vi "SS_fpga_swept_sines.vi"() -> ()   [LabVIEW 2017]
uses:
  controls/boolean_info.ctl
  subVIs/auto-sys-id/controls/sysID_control_params.ctl
  <vilib>/rvi/Emulation/niFpgaGetClockAttributes.vi
  <vilib>/rvi/Emulation/niFpgaSctlEmulationGetInTimedLoop.vi
  <vilib>/rvi/Emulation/niFpgaEmulationReportErrorSimple.vi
  <vilib>/rvi/Emulation/niFpgaCriticalErrorInLSC.vi
  <vilib>/rvi/Emulation/niFpgaProcessEmulError.vi
panel:
  in  "Log-Channel_select":bool[](array[boolean])=[TRUE, TRUE, TRUE, TRUE, FALSE, FALSE]
  in  "Close Loop?":bool
  in  "Nsettle":u32
  in  "reset":bool=TRUE
  out "z-u(k)":sgl
  in  "DDS_params":T1={"Accumulator Increment"=100000, "Phase Shift"=0, "Signal Amplitude (x 2^15)"=32768}
  in  "DAC-select":i16(ring) items=["Mod2/AO0", "Mod2/AO1", "Mod2/AO2", "Mod2/AO3", ""]
  in  "ADC-select":i16(ring) items=["Mod2/AI0", "Mod2/AI1", "Mod2/AI2", "Mod2/AI3", ""]
  in  "ABORT":bool
  in  "Subtract y0?":bool
  in  "Swept-Sines-Control-Settings":T2={"u-max"=0.3, "offset"=0.0, "Ki"=0.001} {"offset" format="%#_4g"; "u-max" format="%#_13g"}
  out "iter":i32
  out "All Done":bool
  in  "TsTicks":u32=1600
  out "boolean \nindicators":T3
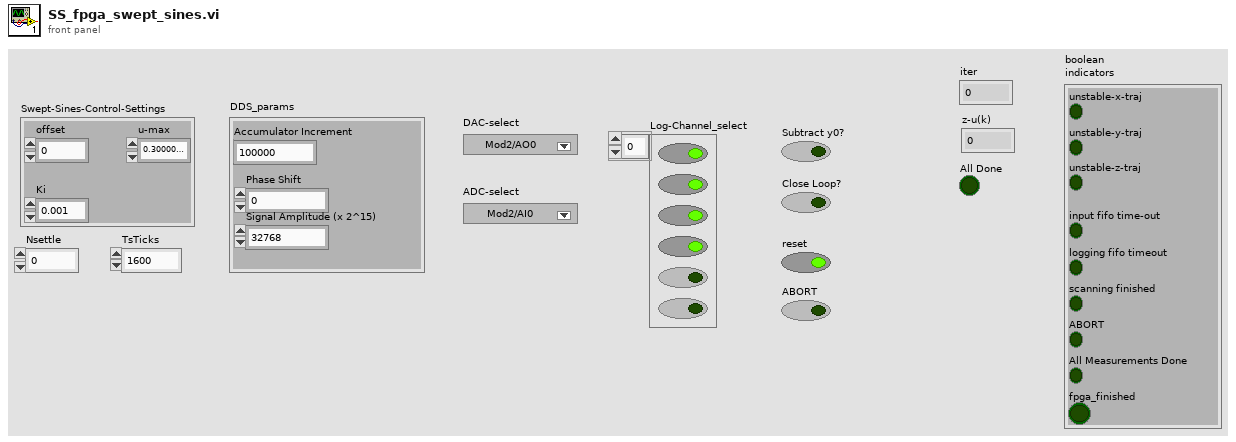
[diagram p1: front panel]
types:
  T1 = cluster{"Accumulator Increment":u32, "Phase Shift":u32, "Signal Amplitude (x 2^15)":u16}
  T2 = typedef "sysID_control_params.ctl" = cluster{"u-max":sgl, "offset":sgl, "Ki":sgl}
  T3 = typedef "boolean_info.ctl" = cluster{"unstable-z-traj":bool, "input fifo time-out":bool, "logging fifo timeout":bool, "scanning finished":bool, "unstable-x-traj":bool, "unstable-y-traj":bool, "ABORT":bool, "All Measurements Done":bool, "fpga_finished":bool}
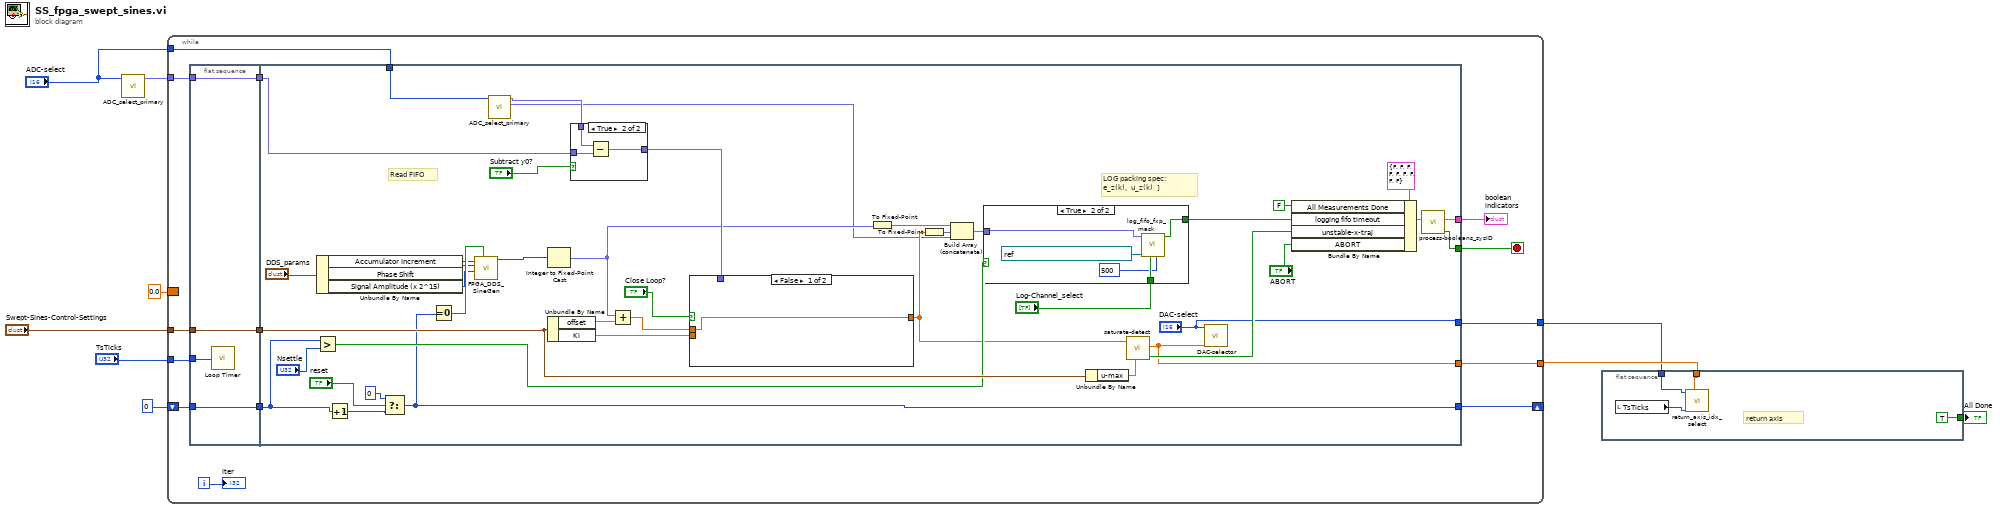
[diagram p0: block diagram]
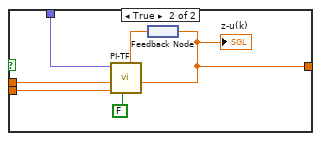
[diagram p2: hidden frame]
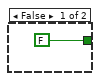
[diagram p4: hidden frame]
diagram:
  n1 = call "ADC_select_primary.vi"("ADC-primary-select"="ADC-select") -> ("Primary-ADC"=w2:fxp<+/-,24,5>)  [unwired: 9 in, 1 out]
  n2 = while {
    tunnel: "Swept-Sines-Control-Settings" -> [w22]
    tunnel: "TsTicks" -> [w21]
    tunnel: [w20] -> w8
    tunnel: "ADC-select" -> [w17]
    shift-right: [w14] -> _
    shift-left: u32 0 -> [w13]
    border: sgl 0.0 ("u(k)") -> [_]
    tunnel: [w12] -> w3
    tunnel: w2 -> [w11]
    i -> [w16]
    stop <- w19 stop-if-true
    n3 = flat-sequence {
      tunnel: w21 -> [w26]
      tunnel: w22 -> [w27]
      tunnel: [w27] -> w23
      tunnel: [w25] -> w15
      tunnel: w13 -> [w25]
      tunnel: w11 -> [w24]
      tunnel: [w24] -> w10
      tunnel: w23 -> [w67]
      tunnel: [w54] -> w20
      tunnel: [w56] -> w19
      tunnel: [w55] -> w18
      tunnel: w17 -> [w30]
      tunnel: w15 -> [w41]
      tunnel: [w40] -> w14
      tunnel: ["DAC-select"] -> w12
      tunnel: w10 -> [w31]
      frame #0 {
        n4 = call "Loop Timer"("Count(Ticks)"=w26) -> ()  [unwired: 1 out]
      }
      frame #1 {
        # "LOG packing spec:\ne_z(k),  u_z(k)  ]"
        # "Read FIFO"
        n5 = Greater?(x=w41, y="Nsettle") -> (0:w46:bool)
        n6 = Unbundle By Name("DDS_params") -> ("Accumulator Increment"=w49:u32, "Phase Shift"=w48:u32, "Signal Amplitude (x 2^15)"=w47:u16)
        n7 = Increment(x=w41) -> (x+1=w45:u32)
        n8 = Select(t=u32 0, s="reset", f=w45) -> (s? t:f=w40:u32)
        n9 = Equal To 0?(x=w40) -> (x = 0?=w50:bool)
        n10 = call "FPGA_DDS_SineGen.vi"("Reset Accumulator"=w50, "Signal Amplitude (x 2^15)"=w47, "Phase Shift"=w48, "Accumulator Increment"=w49) -> ("Signal Value"=w51:i16)  [unwired: 6 in, 1 out]
        n11 = call "ADC_select_primary.vi"("ADC-primary-select"=w30) -> ("ADC-all"=w28:fxp<+/-,24,5>[], "Primary-ADC"=w32:fxp<+/-,24,5>)  [unwired: 9 in]
        n12 = Unbundle By Name(w67) -> ("offset"=w64:sgl, "Ki"=w53:sgl)
        n13 = Integer to Fixed-Point Cast(integer=w51) -> (fixed-point=w34:fxp<+/-,16,5>)  [unwired: 1 in]
        n14 = case shown="True" "Subtract y0?" {
          tunnel: w31 -> [_ w78]
          tunnel: w32 -> [w76 w79]
          tunnel: [w76 w77] -> w52
          frame False {
          }
          frame True {
            n15 = Subtract(x=w79, y=w78) -> (x-y=w77:fxp<+/-,25,6>)
          }
        }
        n16 = Add(x=w34, y=w64) -> (x+y=w65:sgl)
        n17 = case shown="False" "Close Loop?" {
          tunnel: w65 -> [w69 w73]
          tunnel: w53 -> [_ w72]
          tunnel: w52 -> [_ w70]
          tunnel: [w69 w71] -> w36
          frame False {
          }
          frame True {
            n18 = feedback #1() -> (w75:sgl)
            n19 = call "PI-TF.vi"("u(k-1)"=w75, "reset"=FALSE, "Ki"=w72, "setpoint"=w73, "y(k)"=w70) -> ("u(k)"=w71:sgl)  [unwired: 6 in]
            "z-u(k)" <- w71
            n20 = feedback-in #1(w71) -> ()
          }
        }
        n21 = To Fixed-Point(number=w34) -> (fixed-point=w35:fxp<+/-,25,6>)  [unwired: 1 in]
        n22 = To Fixed-Point(number=w36) -> (fixed-point=w29:fxp<+/-,25,6>)  [unwired: 1 in]
        n23 = Build Array (concatenate)(w35, w29, w28) -> (w68:fxp<+/-,25,6>[])
        n24 = case shown="True" w46 {
          tunnel: w68 -> [_ w85]
          tunnel: [FALSE ("logging-timeout?") w84] -> w57
          tunnel: "Log-Channel_select" -> [_ w82]
          frame False {
          }
          frame True {
            n25 = call "log_fifo_fxp_mask.vi"("Timeout(ticks)"=500, "Log-Channel_select"=w82, "FIFO In"=refnum<k21> "fpga-to-host-fxp-16-5", "input-data"=w85) -> ("logging-timeout?"=w84:bool)  [unwired: 7 in]
          }
        }
        n26 = Unbundle By Name(w67) -> ("u-max"=w66:sgl)
        n27 = call "saturate-detect.vi"("bound"=w66, "x"=w36) -> ("saturated"=w58:bool, "sat(x)"=w54:sgl)  [unwired: 8 in]
        n28 = call "DAC-selector.vi"("data-in"=w54, "DAC-select"="DAC-select") -> ()  [unwired: 10 in]
        n29 = Bundle By Name(cluster=T3 {"unstable-z-traj"=FALSE, "input fifo time-out"=FALSE, "logging fifo timeout"=FALSE, "scanning finished"=FALSE, "unstable-x-traj"=FALSE, "unstable-y-traj"=FALSE, "ABORT"=FALSE, "All Measurements Done"=FALSE, "fpga_finished"=FALSE} ("boolean errors"), "All Measurements Done"=FALSE, "logging fifo timeout"=w57, "unstable-x-traj"=w58, "ABORT"="ABORT") -> (w60:T3)
        n30 = call "process-booleans_sysID.vi"("boolean indicators 2"=w60) -> ("scaning finished"=w56:bool, "boolean indicators"=w55:T3)  [unwired: 9 in]
      }
    }
    "boolean \nindicators" <- w18
    "iter" <- w16
  }
  n31 = flat-sequence {
    tunnel: w8 -> [w88]
    tunnel: [TRUE] -> w7
    tunnel: w3 -> [w87]
    frame #0 {
      # "return axis"
      n32 = local read "TsTicks"() -> (w86:u32)
      n33 = call "return_axis_idx_select.vi"("u(0)"=w88, "TsTicks"=w86, "DAC-select"=w87) -> ()  [unwired: 9 in]
    }
  }
  "All Done" <- w7
